vi "Easy2Acquire.ConvertQuat2Euler.vi"(5 "3D Picture":refnum<vi>, 7 "3DRef":refnum<vi>, 10 "GetID":string, 11 "MotionData":dbl[][](array[numeric])) -> (2 "Euler":dbl[][](array[numeric]), 3 "Accel":dbl[][](array[numeric]))   [LabVIEW 2017]
uses:
  <vilib>/picture/3D Picture Control/NI_3D Picture Control.lvlib
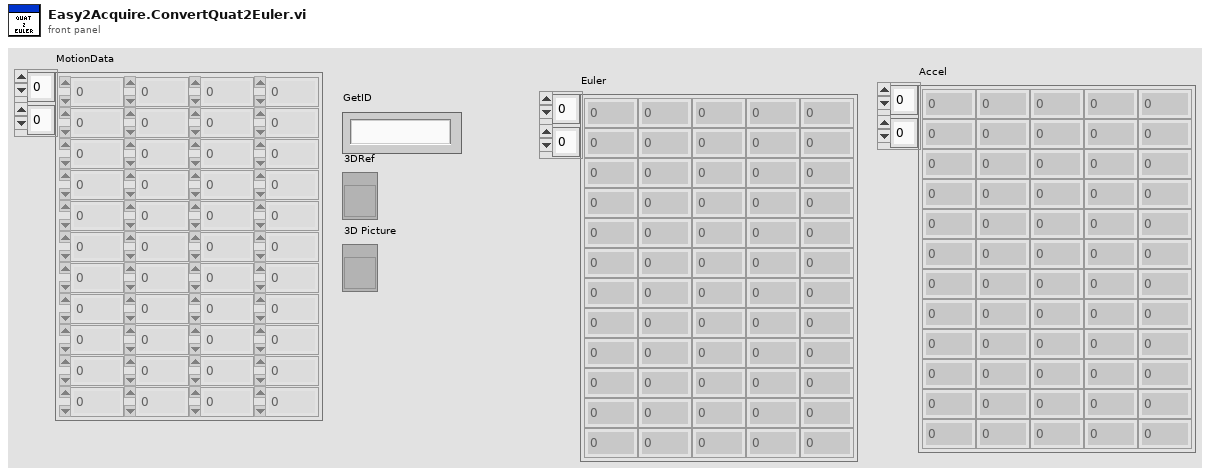
[diagram p1: front panel]
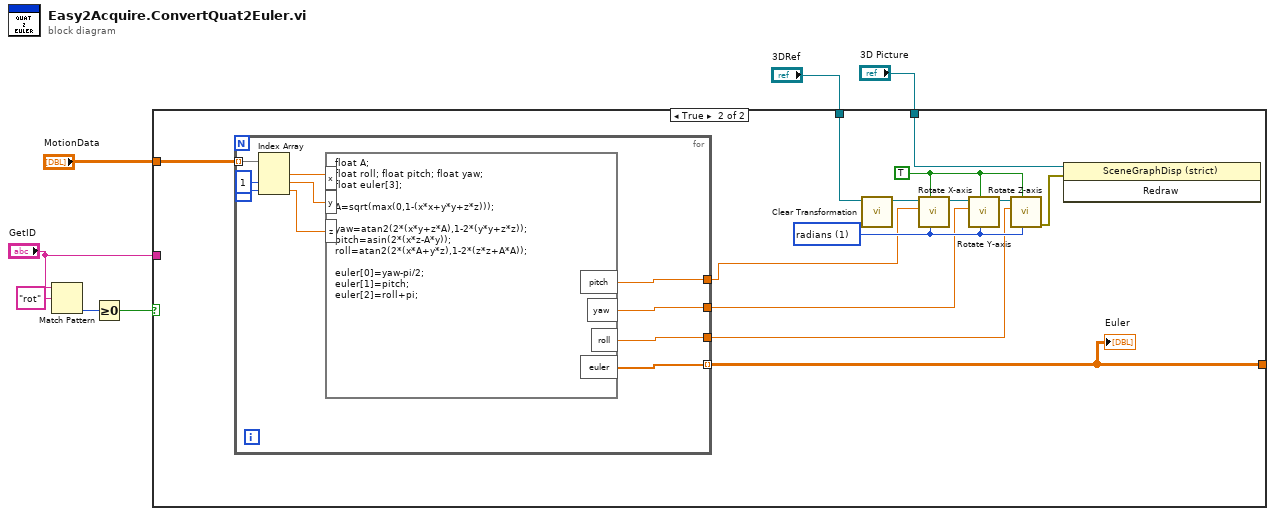
[diagram p0: block diagram]
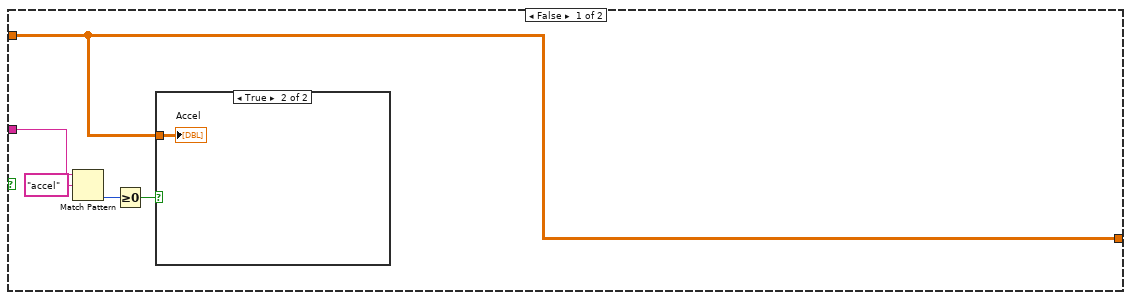
[diagram p2: hidden frame]
diagram:
  n1 = Match Pattern(string="GetID", regular expression="rot") -> (offset past match=w5:i32)  [unwired: 1 in, 3 out]
  n2 = Greater Or Equal To 0?(x=w5) -> (x >= 0?=w6:bool)
  n3 = case shown="True" w6 {
    tunnel: "MotionData" -> [w8 w26]
    tunnel: [w8 w25] -> _
    tunnel: "GetID" -> [w9 _]
    tunnel: "3DRef" -> [_ w17]
    tunnel: "3D Picture" -> [_ w18]
    frame False {
      n4 = Match Pattern(string=w9, regular expression="accel") -> (offset past match=w11:i32)  [unwired: 1 in, 3 out]
      n5 = Greater Or Equal To 0?(x=w11) -> (x >= 0?=w10:bool)
      n6 = case shown="True" w10 {
        tunnel: w8 -> [_ w13]
        frame False {
        }
        frame True {
          "Accel" <- w13
        }
      }
    }
    frame True {
      w20 = TRUE ("Relative?")
      w21 = u16 1 items=["degree", "radians"] ("angle unit")
      n7 = for {
        tunnel: w26 -> [w36] mode=indexing
        tunnel: [w30] -> w25 mode=indexing
        tunnel: [w29] -> w16
        tunnel: [w28] -> w14
        tunnel: [w27] -> w15
        n8 = Index Array(array=w36, index #2=1 ("index"), index #3=2 ("index")) -> (element #1=w33:dbl, element #2=w32:dbl, element #3=w31:dbl)  [unwired: 1 in]
        n9 = formula code="float A;\nfloat roll; float pitch; float yaw;\nfloat euler[3];\n\nA=sqrt(max(0,1-(x*x+y*y+z*z)));\n\nyaw=atan2(2*(x*y+z*A),1-2*(y*y+z*z));\npitch=asin(2*(x*z-A*y));\nroll=atan2(2*(x*A+y*z),1-2*(z*z+A*A));\n\neuler[0]=yaw-pi/2;\neuler[1]=pitch;\neuler[2]=roll+pi;"("x"=w33, "y"=w32, "z"=w31) -> ("euler"=w30:dbl[], "roll"=w28:dbl, "pitch"=w29:dbl, "yaw"=w27:dbl)
      }
      "Euler" <- w25
      n10 = call <vilib>:"Clear Transformation.vi"("Object Refnum In"=w17) -> ("Object Refnum Out"=w22:refnum<vi>)  [unwired: 9 in, 1 out]
      n11 = call <vilib>:"Rotate X-axis.vi"("angle unit"=w21, "Relative?"=w20, "angle"=w16, "Scene Object In"=w22) -> ("Scene Object Out"=w23:refnum<vi>)  [unwired: 6 in, 1 out]
      n12 = call <vilib>:"Rotate Y-axis.vi"("angle unit"=w21, "Relative?"=w20, "angle"=w15, "Scene Object In"=w23) -> ("Scene Object Out"=w24:refnum<vi>)  [unwired: 6 in, 1 out]
      n13 = call <vilib>:"Rotate Z-axis.vi"("angle unit"=w21, "Relative?"=w20, "angle"=w14, "Scene Object In"=w24) -> ("error out"=w19:errorcluster)  [unwired: 6 in, 1 out]
      n14 = invoke class="SceneGraphDisp (strict)" method="Redraw"(reference=w18, error in=w19) -> ()  [unwired: 1 in, 3 out]
    }
  }
